vi "REACTOR__SET_VALVULA.vi"(6 "error in (no error)":errorcluster, 7 "Index":i8) -> (0 "error out":errorcluster, 2 "resulting string 1":string="Mide Bronkhorst 1, mide Alicats 1,  y pausa 1.0s", 3 "Cancelled?":bool)   [LabVIEW 2017]
doc: "Use this template to create a dialog box. This template polls the state of the buttons on the front panel and does not use events. Use the Dialog Using Events template (not available in Base package) to create a dialog box with event handling."
panel:
  in  "VALVULA":bool=TRUE
  in  "PAUSA(s)":dbl=1.0 format="%.1f"
  in  "Cancel":bool
  in  "OK":bool
  # "VALVULA"
  # "Noviembre 2022 V1.0  a-sslcdms"
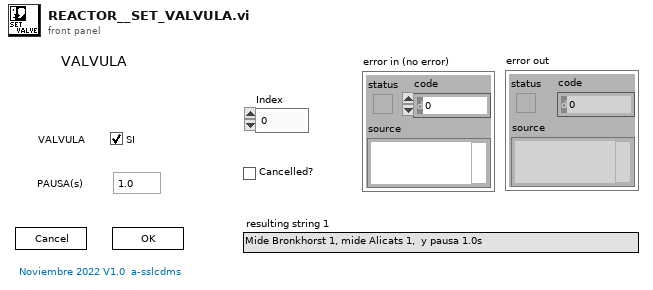
[diagram p1: front panel]
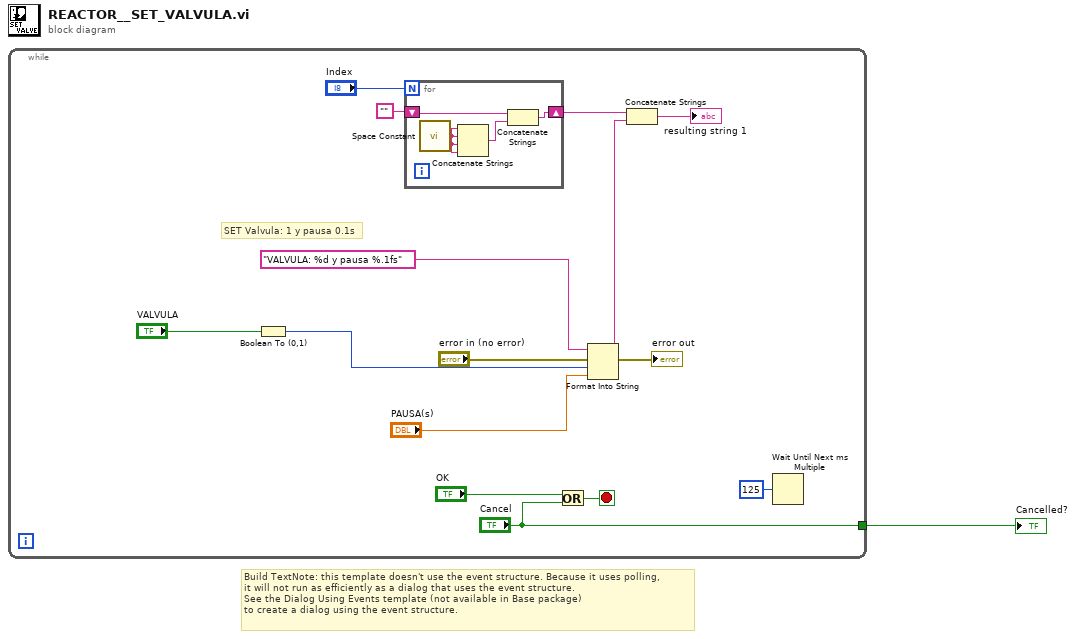
[diagram p0: block diagram]
diagram:
  # "Build TextNote: this template doesn't use the event structure. Because it uses polling, \nit will not run as efficiently as a dialog that uses the event structure.\nSee the Dialog Using Events template (not available in Base package) \nto create a dialog using the event structure."
  n1 = while {
    tunnel: ["Cancel"] -> w1
    stop <- w15 stop-if-true
    # "SET Valvula: 1 y pausa 0.1s"
    n2 = Boolean To (0,1)(Boolean="VALVULA") -> (0, 1=w3:i16)
    n3 = for {
      N: "Index" -> [_]
      shift-right: [w19] -> w7
      shift-left: "" -> [w18]
      n4 = call <vilib>:"Space Constant.vi"() -> ("String"=w17:string)
      n5 = Concatenate Strings(w17, w17, w17, w17) -> (w20:string)
      n6 = Concatenate Strings(w18, w20) -> (w19:string)
    }
    n7 = Or(x="OK", y="Cancel") -> (x .or. y?=w15:bool)
    n8 = Format Into String(format string="VALVULA: %d y pausa %.1fs", error in="error in (no error)", w3, "PAUSA(s)") -> (resulting string=w5:string, error out=→"error out":errorcluster)  [unwired: 1 in]
    n9 = Concatenate Strings(w7, w5) -> (→"resulting string 1":string)
    n10 = Wait Until Next ms Multiple(millisecond multiple=u32 125) -> ()  [unwired: 1 out]
  }
  "Cancelled?" <- w1
